vi "Charts updated.vi"() -> ()   [LabVIEW 2014]
doc: "Es VI te permite explorar de manera basica lo socntroles e indicadores de un programa en Labview."
panel:
  out "Waveform Chart 3":dbl(graph)
  out "Waveform Chart 2":dbl(graph)
  in  "numMin":dbl=100.0
  in  "numMax":dbl
  out "Waveform Chart":dbl(graph)
  in  "stop":bool
  # "Different behaviors for \nwaveform chart - updated"
  # "Strip chart"
  # "Scope chart"
  # "Sweep chart"
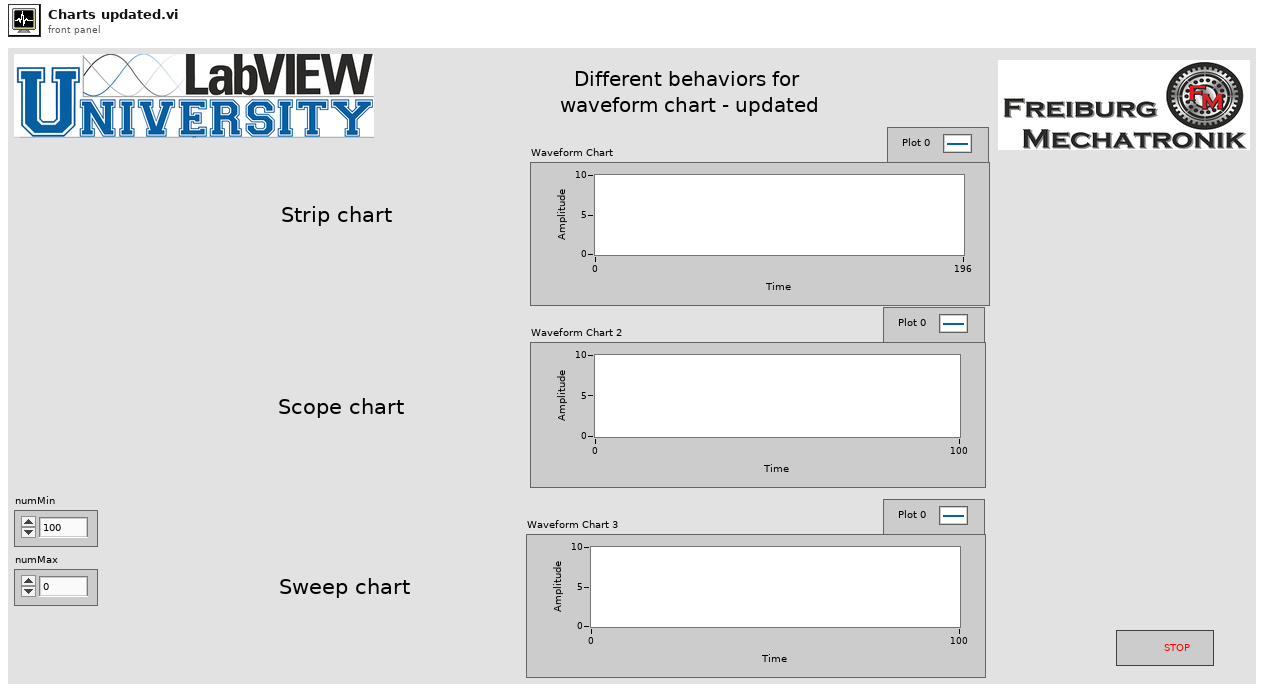
[diagram p1: front panel]
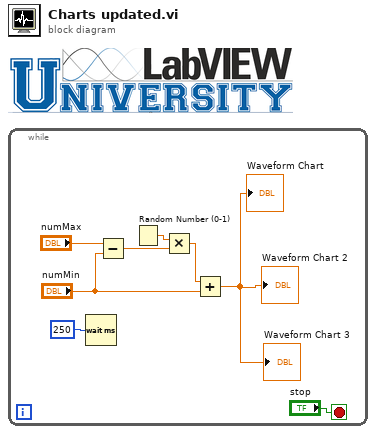
[diagram p0: block diagram]
diagram:
  n1 = while {
    stop <- "stop" stop-if-true
    n2 = Wait (ms)(milliseconds to wait=u32 250) -> ()  [unwired: 1 out]
    n3 = Subtract(x="numMax", y="numMin") -> (x-y=w5:dbl)
    n4 = Random Number (0-1)() -> (number: 0 to 1=w4:dbl)
    n5 = Multiply(x=w4, y=w5) -> (x*y=w7:dbl)
    n6 = Add(x=w7, y="numMin") -> (x+y=→"Waveform Chart" →"Waveform Chart 2" →"Waveform Chart 3":dbl)
  }
